vi "lab session 3.1.vi"(1 "Rupee":dbl) -> (0 "Dollar":dbl)   [LabVIEW 2020]
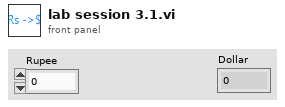
[diagram p1: front panel]
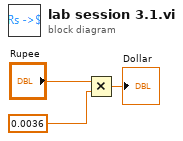
[diagram p0: block diagram]
diagram:
  n1 = Multiply(x="Rupee", y=0.0036) -> (x*y=→"Dollar":dbl)
